vi "Calibrator.vi"(2 "Channels":T26 items=["Dev6/ai0", "Dev6/ai1", "Dev6/ai2", "Dev6/ai3"]) -> (7 "sensor file path":path, 10 "Sensor Names":string[](array[string]))   [LabVIEW 2019]
uses:
  toolbar icons/Save configuration.ctl
  toolbar icons/Save calibration.ctl
  toolbar icons/open configuration.ctl
  toolbar icons/Open calibration.ctl
  toolbar icons/NF90 cal.ctl
  toolbar icons/pH cal.ctl
  toolbar icons/D.O. cal.ctl
  TCP DAQ/Set.ctl
  TCP DAQ/clear offset.ctl
  toolbar icons/Edit calibration.ctl
  toolbar icons/copy sensor.ctl
  toolbar icons/insert sensor.ctl
  toolbar icons/delete sensor.ctl
  DAQ configuration/Sensor array.ctl
  DAQ configuration/channel identifier.ctl
  calibrator graph.ctl
  toolbar icons/help.ctl
  TCP DAQ/Sensor data.ctl
  DAQ configuration/sensor cluster.ctl
  conversion.ctl
  DAQ configuration/scale type.ctl
  correspondence table.ctl
  pH/pH scale.ctl
  Dissolved Oxygen/DO scale.ctl
  Spectrophotometer/Photometer calibration data.ctl
  TCP DAQ/zero.ctl
  Process Controller 3.0/Distributed Daq/Channel config.ctl
  calib array.ctl
  Spectrophotometer/Photometer icon.ctl
  DAQ configuration/Sensor buffer command.ctl
  <vilib>/Platform/browser.llb/Open URL in Default Browser (string).vi
panel:
  in  "Photometer":T1
  out "Channel Config Initial":T2 {"Calibration matrix"."D.O."."K" format="%.6f"; "Calibration matrix"."D.O."."Temperature" format="%.2f"; "Calibration matrix"."pH scale"."Buffers"."V/T" format="%.5f"; "Calibration matrix"."pH scale"."Buffers"."Buffer" format="%.2f"; "Calibration matrix"."pH scale"."Temperature" format="%.2f"; "Calibration matrix"."offset (physical units)" format="%.5f"; "Calibration matrix"."correspondence table"."volts" format="%.4f"; "Calibration matrix"."correspondence table"."physical units" format="%.4f"; "Calibration matrix"."second channel" min=-1; "Calibration matrix"."offset (volts)" format="%.5f"; "Calibration matrix"."conversion matrix" format="%.4e"}
  out "number of available channels":u16
  in  "Zero":T11
  in  "Sensor List":i32(listbox)=-1
  in  "Save configuration":T12
  in  "Save calibration":T13
  in  "Open configuration":T14
  in  "Open calibration":T15
  in  "units":string
  in  "name":string
  in  "nf90":T16
  in  "pH":T17
  in  "DO":T18
  in  "Set clear":T21 {"target value" format="%.1p"}
  in  "Edit calibration":T22
  in  "Cancel":bool
  in  "Duplicate Sensor":T23
  in  "Add Sensor":T24
  in  "Delete Sensor":T25
  in  "OK":bool
  in  "data rate (ms)":u32=10
  in  "history length":u16=100 min=1
  out "Data Display":T27 {"average data rate (Hz)" format="%.2f"; "Min Voltage" format="%.3f"; "Max Voltage" format="%.3f"; "Mean (Volts)" format="%.5f"; "Mean (scaled)" format="%.2f"}
  in  "Volts":T5={"conversion matrix"=[[0.0, 0.0], [0.0, 0.0], [0.0, 0.0], [0.0, 0.0], [0.0, 0.0], [0.0, 0.0]], "units"="volts", "name"="", "scale type"=enum."Volts", "offset (volts)"=0.0, "second channel"=0, "correspondence table"=[], "offset (physical units)"=0.0, "pH scale"={"Buffers"=[], "Temperature"=0.0}, "D.O."={"Temperature"=0.0, "K"=0.0, "barometric pressure"=0.0}, "Photometer data"={"Dark Voltage"=0.0, "Blank Voltage"=0.0, "Standards"=[]}} {"D.O."."K" format="%.6f"; "D.O."."Temperature" format="%.2f"; "pH scale"."Buffers"."V/T" format="%.5f"; "pH scale"."Buffers"."Buffer" format="%.2f"; "pH scale"."Temperature" format="%.2f"; "offset (physical units)" format="%.5f"; "correspondence table"."volts" format="%.4f"; "correspondence table"."physical units" format="%.4f"; "second channel" min=-1; "offset (volts)" format="%.5f"; "conversion matrix" format="%.4e"}
  out "Initial Ports":T26
  out "Sensor Data":T28 {"Sensor array"."scaled" format="%.2f"; "Sensor array"."voltage" format="%.4f"; "Time" format="%<%I:%M:%S%2u %p\n%m/%d/%Y>T"}
  in  "Help":T30
  in  "stop":bool
  # "C"
  # "kPa"
  # "C"
  # "V"
  # "V"
  # "C"
  # "kPa"
  # "C"
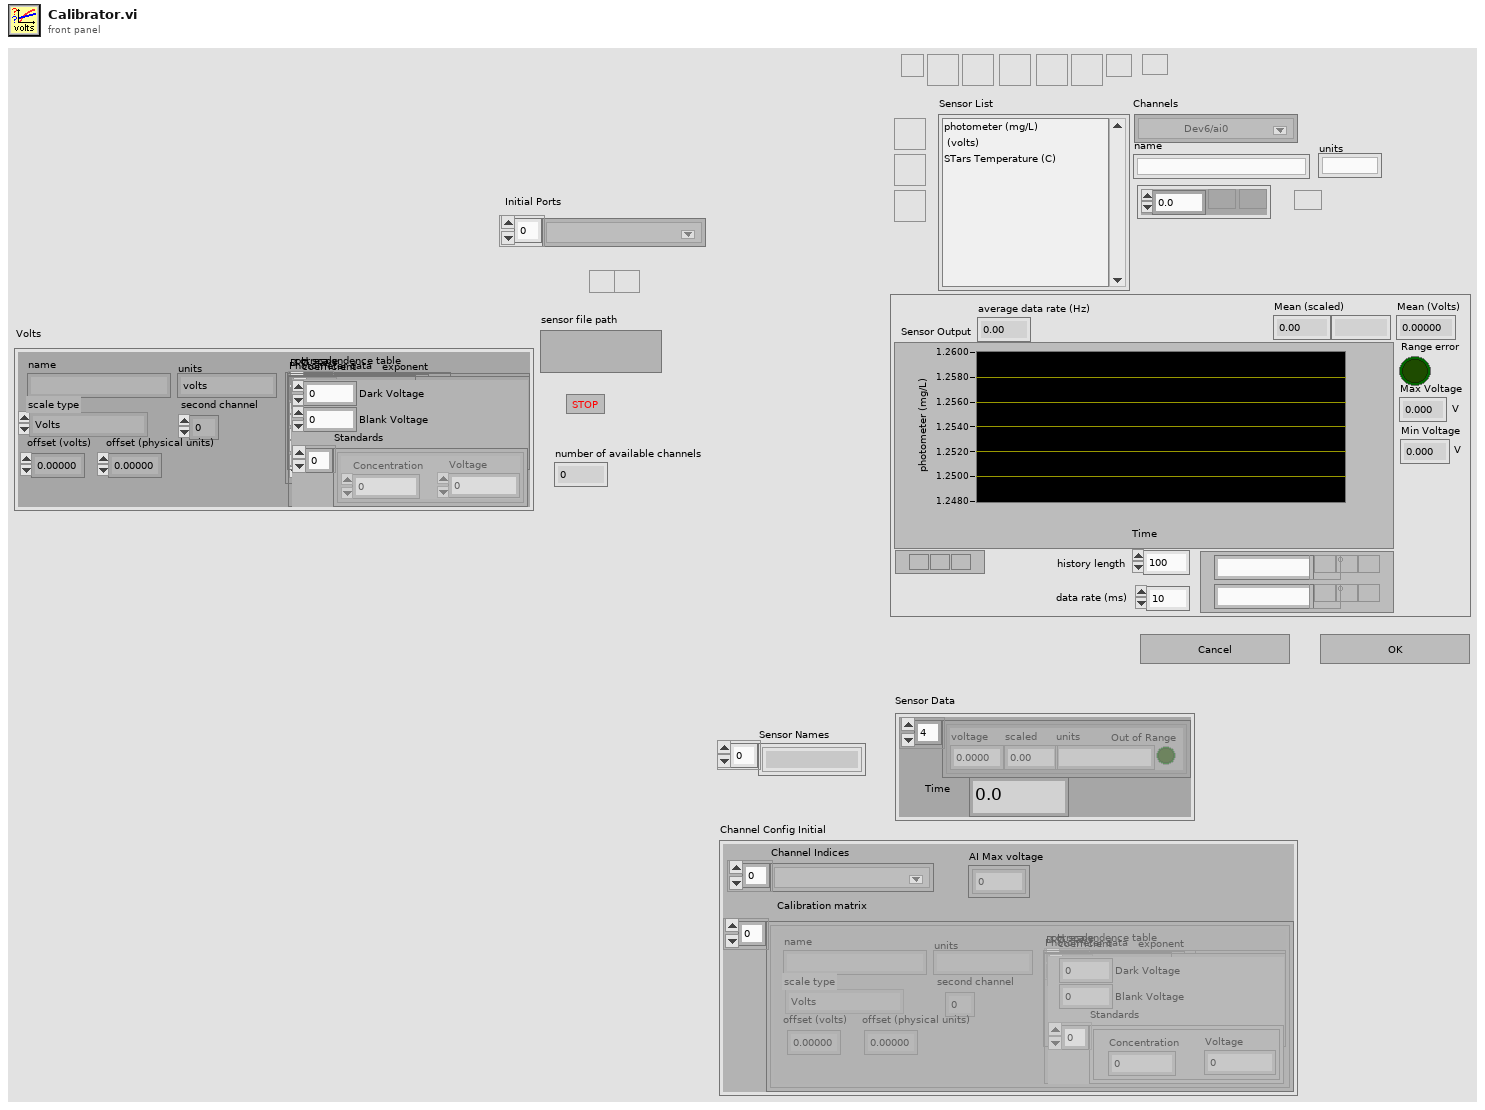
[diagram p1: front panel]
types:
  T1 = typedef "Photometer icon.ctl" = bool
  T2 = typedef "Channel config.ctl" = cluster{"Channel Indices":T3[], "AI Max voltage":dbl[], "Calibration matrix":T4}
  T3 = typedef "channel identifier.ctl" = u16
  T4 = typedef "calib array.ctl" = T5[]
  T5 = typedef "conversion.ctl" = cluster{"conversion matrix":sgl[][], "units":string, "name":string, "scale type":T6, "offset (volts)":dbl, "second channel":i8, "correspondence table":T7, "offset (physical units)":dbl, "pH scale":T8, "D.O.":T9, "Photometer data":T10}
  T6 = typedef "scale type.ctl" = enum16{"Volts", "Polynomial", "Correspondence Table", "pH", "Dissolved Oxygen", "Quadratic", "Photometer"}
  T7 = typedef "correspondence table.ctl" = cluster{"physical units":dbl, "volts":dbl}[]
  T8 = typedef "pH scale.ctl" = cluster{"Buffers":cluster{"Buffer":dbl, "Calibrated":bool, "V/T":dbl}[], "Temperature":dbl}
  T9 = typedef "DO scale.ctl" = cluster{"Temperature":dbl, "K":dbl, "barometric pressure":dbl}
  T10 = typedef "Photometer calibration data.ctl" = cluster{"Dark Voltage":dbl, "Blank Voltage":dbl, "Standards":cluster{"Concentration":dbl, "Voltage":dbl}[]}
  T11 = typedef "zero.ctl" = bool
  T12 = typedef "Save configuration.ctl" = bool
  T13 = typedef "Save calibration.ctl" = bool
  T14 = typedef "open configuration.ctl" = bool
  T15 = typedef "Open calibration.ctl" = bool
  T16 = typedef "NF90 cal.ctl" = bool
  T17 = typedef "pH cal.ctl" = bool
  T18 = typedef "D.O. cal.ctl" = bool
  T19 = typedef "Set.ctl" = bool
  T20 = typedef "clear offset.ctl" = bool
  T21 = cluster{"Set":T19, "target value":dbl, "Clear":T20}
  T22 = typedef "Edit calibration.ctl" = bool
  T23 = typedef "copy sensor.ctl" = bool
  T24 = typedef "insert sensor.ctl" = bool
  T25 = typedef "delete sensor.ctl" = bool
  T26 = typedef "Sensor array.ctl" = T3[]
  T27 = typedef "calibrator graph.ctl" = cluster{"Range error":bool, "Mean (scaled)":dbl, "Mean (Volts)":dbl, "Max Voltage":dbl, "Min Voltage":dbl, "units":string, "Sensor Output":cluster{dbl[], dbl[]}[], "average data rate (Hz)":dbl}
  T28 = typedef "Sensor data.ctl" = cluster{" Sensor array":T29[], "Time":dbl}
  T29 = typedef "sensor cluster.ctl" = cluster{"voltage":sgl, "scaled":sgl, "units":string, "Out of Range":bool}
  T30 = typedef "help.ctl" = bool
  T31 = typedef "Sensor buffer command.ctl" = enum16{"read average", "read recent", "read all", "write", "set buffer size", "Read channel config", "Write channel config", "clear"}
  T32 = enum8{"Enabled", "Disabled", "Disabled and Grayed Out"}
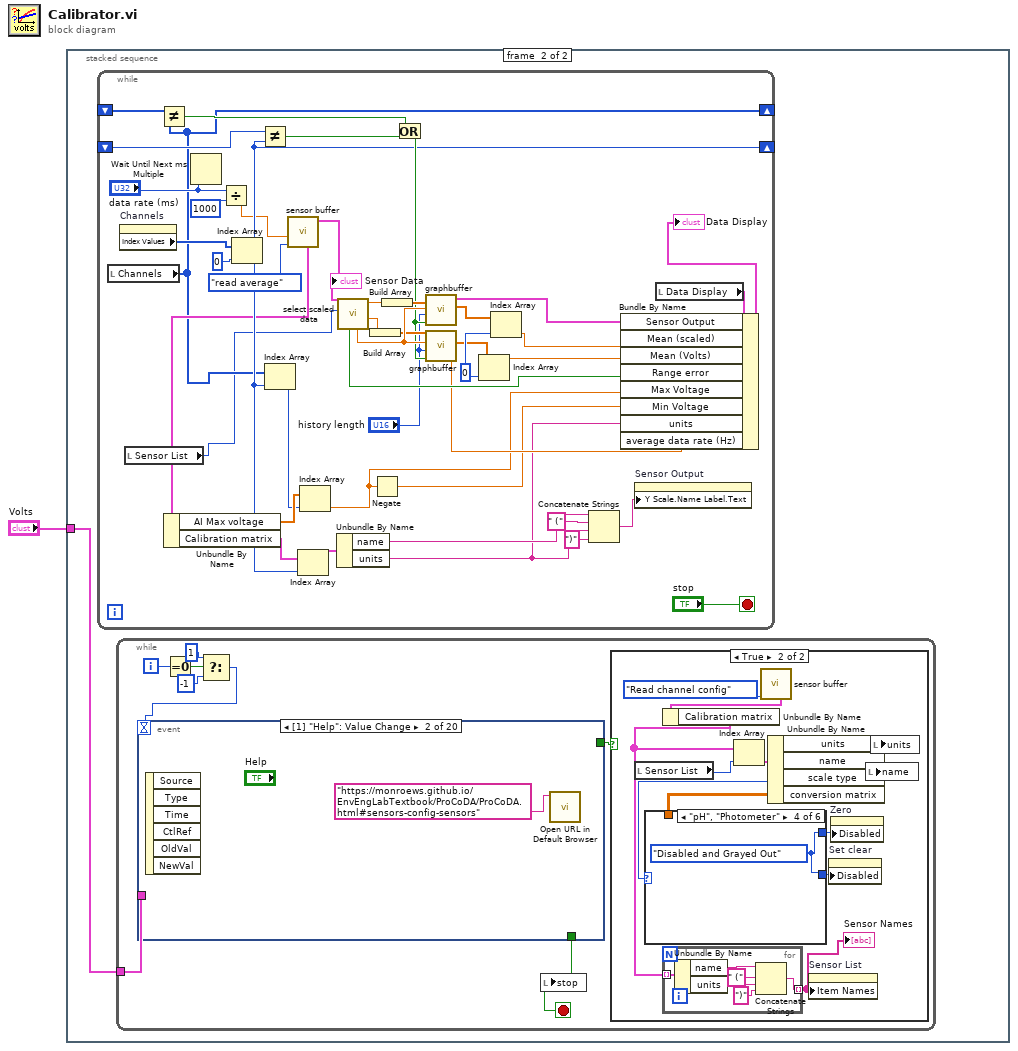
[diagram p0: block diagram]
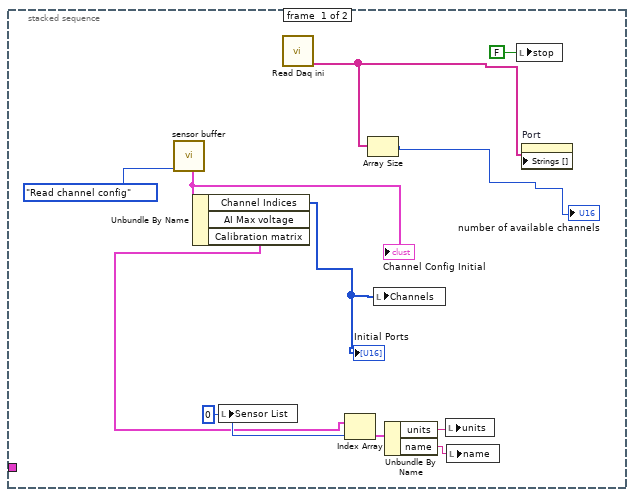
[diagram p2: hidden frame]
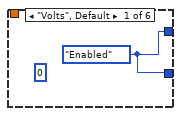
[diagram p4: hidden frame]
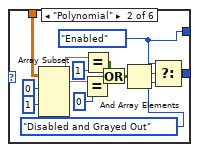
[diagram p5: hidden frame]
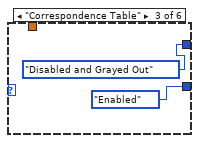
[diagram p6: hidden frame]
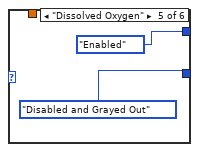
[diagram p7: hidden frame]
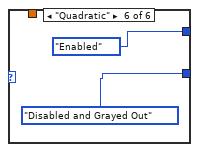
[diagram p8: hidden frame]
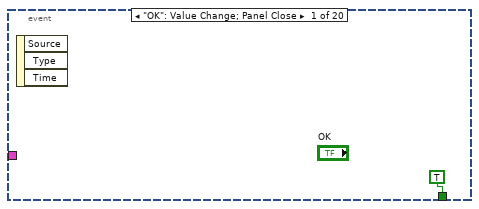
[diagram p9: hidden frame]
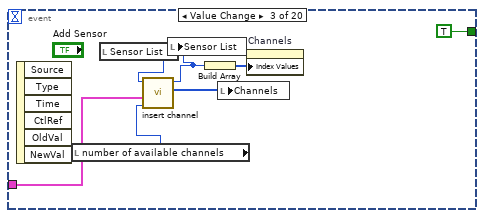
[diagram p10: hidden frame]
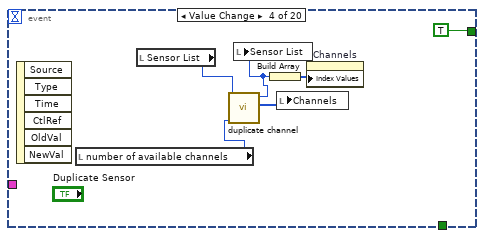
[diagram p11: hidden frame]
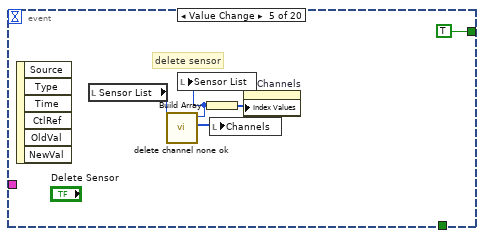
[diagram p12: hidden frame]
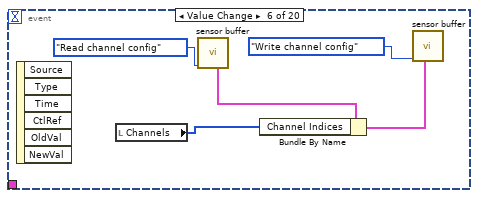
[diagram p13: hidden frame]
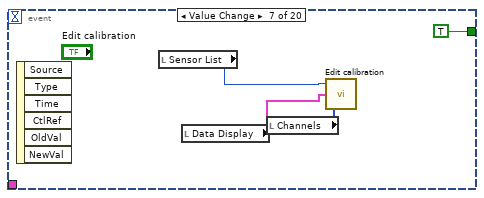
[diagram p14: hidden frame]
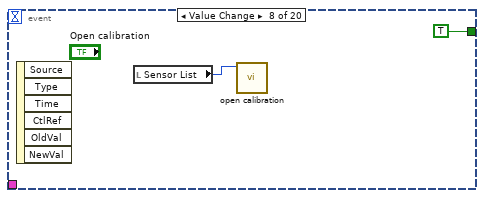
[diagram p15: hidden frame]
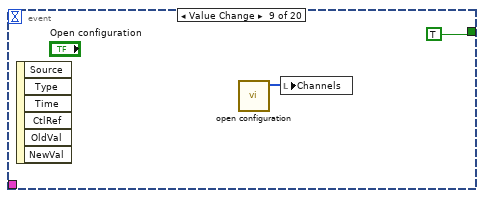
[diagram p16: hidden frame]
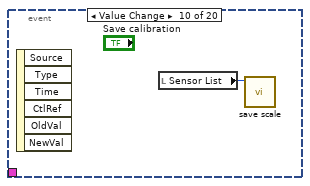
[diagram p17: hidden frame]
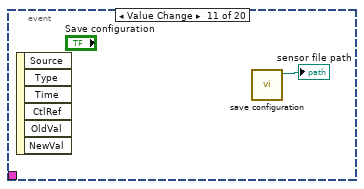
[diagram p18: hidden frame]
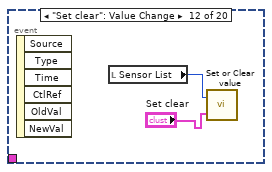
[diagram p19: hidden frame]
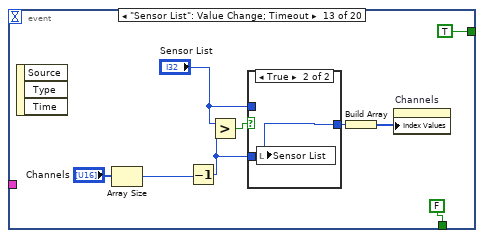
[diagram p20: hidden frame]
diagram:
  n1 = stacked-sequence {
    tunnel: "Volts" -> [_ w13]
    frame #0 {
      w5 = u32 0 ("Index")
      n2 = call "sensor buffer.vi"("command"=Sensor_buffer_command."Read channel config") -> ("Channel Config out"=w9:T2)  [unwired: 6 in, 4 out]
      "Channel Config Initial" <- w9
      n3 = Unbundle By Name(w9) -> ("Channel Indices"=w3:T3[], "Calibration matrix"=w4:T4)  [unwired: 1 out]
      "Initial Ports" <- w3
      n4 = local write "Sensor List"(w5) -> ()
      n5 = call "Read Daq ini.vi"() -> ("AI Channels"=w11:string[])  [unwired: 3 in, 8 out]
      n6 = Index Array(array=w4, index=w5) -> (element=w6:T5)
      n7 = Array Size(array=w11) -> (size(s)=→"number of available channels":i32)
      n8 = local write "Channels"(w3) -> ()
      n9 = Unbundle By Name(w6) -> ("units"=w7:string, "name"=w8:string)
      n10 = local write "units"(w7) -> ()
      n11 = local write "name"(w8) -> ()
      n12 = local write "stop"(FALSE ("stop")) -> ()
      n13 = property on="Port" class="Ring (strict)"("Strings []"=w11) -> ()  [unwired: 2 in, 2 out]
    }
    frame #1 {
      n14 = while {
        shift-left: _ -> [w47]
        shift-right: [w27] -> _
        shift-left: _ -> [w48]
        shift-right: [w16] -> _
        stop <- "stop" stop-if-true
        w55 = 0 ("Index")
        n15 = local read "Channels"() -> (w16:T26)
        n16 = property on="Channels" class="Arr (strict)"() -> ("Index Values"=w33:u32[])  [unwired: 2 in, 2 out]
        n17 = local read "Sensor List"() -> (w14:i32)
        n18 = Not Equal?(x=w48, y=w16) -> (x != y?=w46:bool)
        n19 = Wait Until Next ms Multiple(millisecond multiple="data rate (ms)") -> ()  [unwired: 1 out]
        n20 = Divide(x="data rate (ms)", y=u32 1000) -> (x/y=w19:dbl)
        n21 = Index Array(array=w33, index=0 ("Index")) -> (element=w27:u32)
        n22 = Not Equal?(x=w47, y=w27) -> (x != y?=w45:bool)
        n23 = Index Array(array=w16, index=w27) -> (element=w15:T3)
        n24 = call "sensor buffer.vi"("command"=Sensor_buffer_command."read average", "smooth interval (s)"=w19) -> ("Calibrated data"=w25:T28, "Channel Config out"=w24:T2)  [unwired: 5 in, 3 out]
        "Sensor Data" <- w25
        n25 = Unbundle By Name(w24) -> ("AI Max voltage"=w22:dbl[], "Calibration matrix"=w23:T4)
        n26 = Index Array(array=w23, index=w27) -> (element=w44:T5)
        n27 = Index Array(array=w22, index=w15) -> (element=w21:dbl)
        n28 = Unbundle By Name(w44) -> ("name"=w32:string, "units"=w30:string)
        n29 = call "select scaled data.vi"("Sensor index"=w14, "Sensor Data"=w25) -> ("voltage"=w51:sgl, "scaled"=w57:sgl, "Time"=w52:dbl, "Out of Range"=w39:bool)  [unwired: 4 in, 2 out]
        n30 = Build Array(w51) -> (w50:sgl[])
        n31 = Negate(x=w21) -> (-x=w20:dbl)
        n32 = Build Array(w57) -> (w56:sgl[])
        n33 = Or(x=w46, y=w45) -> (x .or. y?=w37:bool)
        n34 = call "graphbuffer.vi"("Reset"=w37, "history length"="history length", "Time"=w52, "data"=w56) -> ("Mean"=w49:dbl[], "Multiplot graph data"=w42:cluster{dbl[], dbl[]}[])  [unwired: 5 in, 1 out]
        n35 = call "graphbuffer.vi"("Reset"=w37, "history length"="history length", "Time"=w52, "data"=w50) -> ("data rate (Hz)"=w38:dbl, "Mean"=w53:dbl[])  [unwired: 5 in, 1 out]
        n36 = Index Array(array=w53, index=w55) -> (element=w40:dbl)
        n37 = Index Array(array=w49, index=w55) -> (element=w41:dbl)
        n38 = Concatenate Strings(w32, " (" ("string"), w30, ")" ("string")) -> (w28:string)
        n39 = property on="Sensor Output" class="XYGraph (strict)"("Y Scale.Name Label.Text"=w28) -> ()  [unwired: 2 in, 2 out]
        n40 = local read "Data Display"() -> (w43:T27)
        n41 = Bundle By Name(cluster=w43, "Sensor Output"=w42, "Mean (scaled)"=w41, "Mean (Volts)"=w40, "Range error"=w39, "Max Voltage"=w21, "Min Voltage"=w20, "units"=w30, "average data rate (Hz)"=w38) -> (→"Data Display":T27)
      }
      n42 = while {
        tunnel: w13 -> [w65]
        i -> [w63]
        stop <- w58 stop-if-true
        n43 = Equal To 0?(x=w63) -> (x = 0?=w62:bool)
        n44 = Select(t=1, s=w62, f=-1) -> (s? t:f=w59:i32)
        n45 = event shown="[1] \"Help\": Value Change" {
          selector: _ -> [_ _ _ _ _ _ _ _ _ _ _ _ _ _ _ _ _ _ _ _]
          dyn-events: _ -> [_ _ _ _ _ _ _ _ _ _ _ _ _ _ _ _ _ _ _ _]
          timeout: w59 -> [_ _ _ _ _ _ _ _ _ _ _ _ _ _ _ _ _ _ _ _]
          tunnel: [TRUE ("Cancel") _ _ _ _ _ _ _ _ _ _ _ FALSE ("Cancel") _ _ _ _ _ "Cancel" _] -> w58
          tunnel: w65 -> [_ _ w112 _ _ _ _ _ _ _ _ _ _ _ _ _ _ _ _ _]
          tunnel: [_ _ TRUE TRUE TRUE _ TRUE TRUE TRUE _ _ _ TRUE TRUE TRUE TRUE TRUE TRUE TRUE _] -> w64
          event "OK": Value Change; Panel Close {
            n46 = event-data() -> ()  [unwired: 1 in, 3 out]
          }
          event Value Change {
            n47 = event-data() -> ()  [unwired: 1 in, 6 out]
            n48 = call-poly <vilib>:"Open URL in Default Browser.vi"("URL"="https://monroews.github.io/EnvEngLabTextbook/ProCoDA/ProCoDA.html#sensors-config-sensors") -> ()  [unwired: 5 in, 2 out]
          }
          event Value Change {
            n49 = event-data() -> ()  [unwired: 1 in, 6 out]
            n50 = local read "number of available channels"() -> (w107:u16)
            n51 = local read "Sensor List"() -> (w110:i32)
            n52 = call "insert channel.vi"("number of available channels"=w107, "Volts"=w112, "Index"=w110) -> ("Sensor Array out"=w113:T26, "Index out"=w111:u32)  [unwired: 7 in]
            n53 = local write "Sensor List"(w111) -> ()
            n54 = Build Array(w111) -> (w109:u32[])
            n55 = local write "Channels"(w113) -> ()
            n56 = property on="Channels" class="Arr (strict)"("Index Values"=w109) -> ()  [unwired: 2 in, 2 out]
          }
          event Value Change {
            n57 = event-data() -> ()  [unwired: 1 in, 6 out]
            n58 = local read "number of available channels"() -> (w114:u16)
            n59 = local read "Sensor List"() -> (w117:i32)
            n60 = call "duplicate channel.vi"("number of available channels"=w114, "Sensor List"=w117) -> ("Sensor Array out"=w118:T26, "IndexVals"=w116:u32)  [unwired: 8 in]
            n61 = local write "Sensor List"(w116) -> ()
            n62 = Build Array(w116) -> (w119:u32[])
            n63 = local write "Channels"(w118) -> ()
            n64 = property on="Channels" class="Arr (strict)"("Index Values"=w119) -> ()  [unwired: 2 in, 2 out]
          }
          event Value Change {
            # "delete sensor"
            n65 = event-data() -> ()  [unwired: 1 in, 6 out]
            n66 = local read "Sensor List"() -> (w122:i32)
            n67 = call "delete channel none ok.vi"("Indexvals in"=w122) -> ("Sensor Array out"=w123:T26, "Indexvals out"=w121:u32)  [unwired: 9 in]
            n68 = local write "Sensor List"(w121) -> ()
            n69 = Build Array(w121) -> (w124:u32[])
            n70 = local write "Channels"(w123) -> ()
            n71 = property on="Channels" class="Arr (strict)"("Index Values"=w124) -> ()  [unwired: 2 in, 2 out]
          }
          event Value Change {
            n72 = event-data() -> ()  [unwired: 1 in, 6 out]
            n73 = local read "Channels"() -> (w126:T26)
            n74 = call "sensor buffer.vi"("command"=Sensor_buffer_command."Read channel config") -> ("Channel Config out"=w127:T2)  [unwired: 6 in, 4 out]
            n75 = Bundle By Name(cluster=w127, "Channel Indices"=w126) -> (w125:T2)
            n76 = call "sensor buffer.vi"("Channel Config"=w125, "command"=Sensor_buffer_command."Write channel config") -> ()  [unwired: 5 in, 5 out]
          }
          event Value Change {
            n77 = event-data() -> ()  [unwired: 1 in, 6 out]
            n78 = local read "Sensor List"() -> (w133:i32)
            n79 = local read "Data Display"() -> (w132:T27)
            n80 = local read "Channels"() -> (w131:T26)
            n81 = call "Edit calibration.vi"("Ports"=w131, "Data Display"=w132, "Index"=w133) -> ()  [unwired: 2 in]
          }
          event Value Change {
            n82 = event-data() -> ()  [unwired: 1 in, 6 out]
            n83 = local read "Sensor List"() -> (w135:i32)
            n84 = call "open calibration.vi"("Index"=w135) -> ()  [unwired: 8 in, 3 out]
          }
          event Value Change {
            n85 = event-data() -> ()  [unwired: 1 in, 6 out]
            n86 = call "open configuration.vi"() -> ("Channel Indices"=w137:T3[])  [unwired: 6 in, 1 out]
            n87 = local write "Channels"(w137) -> ()
          }
          event Value Change {
            n88 = event-data() -> ()  [unwired: 1 in, 6 out]
            n89 = local read "Sensor List"() -> (w138:i32)
            n90 = call "save scale.vi"("Index"=w138) -> ()  [unwired: 9 in, 1 out]
          }
          event Value Change {
            n91 = event-data() -> ()  [unwired: 1 in, 6 out]
            n92 = call "save configuration.vi"() -> ("sensor file path"=→"sensor file path":path)  [unwired: 6 in, 1 out]
          }
          event "Set clear": Value Change {
            n93 = event-data() -> ()  [unwired: 1 in, 6 out]
            n94 = local read "Sensor List"() -> (w140:i32)
            n95 = call "Set or Clear value.vi"("Set clear"="Set clear", "Index"=w140) -> ()  [unwired: 2 in]
          }
          event "Sensor List": Value Change; Timeout {
            n96 = event-data() -> ()  [unwired: 1 in, 3 out]
            n97 = Array Size(array="Channels") -> (size(s)=w148:i32)
            n98 = Decrement(x=w148) -> (x-1=w146:i32)
            n99 = Greater?(x="Sensor List", y=w146) -> (0:w145:bool)
            n100 = case shown="True" w145 {
              tunnel: [w151 w152] -> w147
              tunnel: "Sensor List" -> [w151 _]
              tunnel: w146 -> [_ w152]
              frame False {
              }
              frame True {
                n101 = local write "Sensor List"(w152) -> ()
              }
            }
            n102 = Build Array(w147) -> (w144:i32[])
            n103 = property on="Channels" class="Arr (strict)"("Index Values"=w144) -> ()  [unwired: 2 in, 2 out]
          }
          event "units", "name": Value Change {
            n104 = event-data() -> ()  [unwired: 1 in, 6 out]
            n105 = local read "Sensor List"() -> (w164:i32)
            n106 = call "sensor buffer.vi"("command"=Sensor_buffer_command."Read channel config") -> ("Channel Config out"=w155:T2)  [unwired: 6 in, 4 out]
            n107 = Unbundle By Name(w155) -> ("Calibration matrix"=w157:T4)
            n108 = Index Array(array=w157, index=w164) -> (element=w163:T5)
            n109 = Bundle By Name(cluster=w163, "units"="units", "name"="name") -> (w162:T5)
            n110 = Replace Array Subset(array=w157, new element=w162, index=w164) -> (w154:T4)
            n111 = Bundle By Name(cluster=w155, "Calibration matrix"=w154) -> (w153:T2)
            n112 = call "sensor buffer.vi"("Channel Config"=w153, "command"=Sensor_buffer_command."Write channel config") -> ()  [unwired: 5 in, 5 out]
          }
          event Value Change {
            n113 = event-data() -> ()  [unwired: 1 in, 6 out]
            n114 = local read "Sensor List"() -> (w166:i32)
            n115 = call "calibrate DO.vi"("Index"=w166) -> ()  [unwired: 11 in]
          }
          event Value Change {
            n116 = event-data() -> ()  [unwired: 1 in, 6 out]
            n117 = local read "Sensor List"() -> (w167:i32)
            n118 = call "pH Meter.vi"("pH index"=w167) -> ()  [unwired: 11 in]
          }
          event Value Change {
            n119 = event-data() -> ()  [unwired: 1 in, 6 out]
            n120 = local read "Sensor List"() -> (w170:i32)
            n121 = call "Photometer calibration.vi"("Photometer index"=w170) -> ()  [unwired: 11 in]
          }
          event Value Change {
            n122 = event-data() -> ()  [unwired: 1 in, 6 out]
            n123 = local read "Sensor List"() -> (w172:i32)
            n124 = local read "Channels"() -> (w173:T26)
            n125 = call "NF90 calibrator.vi"("Ports"=w173, "channel index"=w172) -> ()  [unwired: 10 in]
          }
          event "Cancel": Value Change {
            n126 = event-data() -> ()  [unwired: 1 in, 6 out]
            n127 = local read "Channel Config Initial"() -> (w175:T2)
            n128 = call "sensor buffer.vi"("Channel Config"=w175, "command"=Sensor_buffer_command."Write channel config") -> ()  [unwired: 5 in, 5 out]
          }
          event Value Change {
            n129 = event-data() -> ()  [unwired: 1 in, 6 out]
            n130 = call "sensor buffer.vi"("command"=Sensor_buffer_command."read average", "smooth interval (s)"=sgl 5.0) -> ("Calibrated data"=w178:T28)  [unwired: 5 in, 4 out]
            n131 = local read "Sensor List"() -> (w182:i32)
            n132 = call "select scaled data.vi"("Sensor index"=w182, "Sensor Data"=w178) -> ("voltage"=w181:sgl)  [unwired: 4 in, 5 out]
            n133 = call "zero channel.vi"("Index"=w182, "Mean (Volts)"=w181) -> ()  [unwired: 6 in]
          }
        }
        n134 = local write "stop"(w58) -> ()
        n135 = case shown="True" w64 {
          frame False {
          }
          frame True {
            n136 = local read "Sensor List"() -> (w74:i32)
            n137 = call "sensor buffer.vi"("command"=Sensor_buffer_command."Read channel config") -> ("Channel Config out"=w68:T2)  [unwired: 6 in, 4 out]
            n138 = Unbundle By Name(w68) -> ("Calibration matrix"=w67:T4)
            n139 = for {
              tunnel: w67 -> [w104] mode=indexing
              tunnel: [w99] -> w71 mode=indexing
              n140 = Unbundle By Name(w104) -> ("name"=w103:string, "units"=w101:string)
              n141 = Concatenate Strings(w103, " (" ("string"), w101, ")" ("string")) -> (w99:string)
            }
            "Sensor Names" <- w71
            n142 = Index Array(array=w67, index=w74) -> (element=w75:T5)
            n143 = Unbundle By Name(w75) -> ("units"=w77:string, "name"=w76:string, "scale type"=w73:T6, "conversion matrix"=w66:sgl[][])
            n144 = case shown="\"pH\", \"Photometer\"" w73 {
              tunnel: [w78 w81 T32."Enabled" ("Disabled") w94 T32."Disabled and Grayed Out" ("Disabled") T32."Disabled and Grayed Out" ("Disabled")] -> w72
              tunnel: w66 -> [_ w91 _ _ _ _]
              tunnel: [w78 w79 T32."Disabled and Grayed Out" ("Disabled") w94 T32."Enabled" ("Disabled") T32."Enabled" ("Disabled")] -> w70
              frame "Volts", Default {
                w78 = T32."Enabled" ("Disabled")
                (unwired) u8 0 ("Disabled")
              }
              frame "Polynomial" {
                w79 = T32."Enabled" ("Disabled")
                n145 = Array Subset(array=w91, index (row)=0 ("index"), index (col)=1 ("index")) -> (w86:sgl[][])  [unwired: 2 in]
                n146 = Equal?(x=w86, y=u8 0 ("Disabled")) -> (x = y?=w84:bool[][])
                n147 = Equal?(x=w86, y=u8 1 ("Disabled")) -> (x = y?=w85:bool[][])
                n148 = Or(x=w85, y=w84) -> (x .or. y?=w83:bool[][])
                n149 = And Array Elements(Boolean array=w83) -> (logical AND=w82:bool)
                n150 = Select(t=w79, s=w82, f=T32."Disabled and Grayed Out" ("Disabled")) -> (s? t:f=w81:T32)
              }
              frame "Correspondence Table" {
              }
              frame "pH", "Photometer" {
                w94 = T32."Disabled and Grayed Out" ("Disabled")
              }
              frame "Dissolved Oxygen" {
              }
              frame "Quadratic" {
              }
            }
            n151 = property on="Sensor List" class="LstBox (strict)"("Item Names"=w71) -> ()  [unwired: 2 in, 2 out]
            n152 = property on="Set clear" class="Clust"("Disabled"=w72) -> ()  [unwired: 2 in, 2 out]
            n153 = property on="Zero" class="Bool"("Disabled"=w70) -> ()  [unwired: 2 in, 2 out]
            n154 = local write "name"(w76) -> ()
            n155 = local write "units"(w77) -> ()
          }
        }
      }
    }
  }
